vi "cumplimiento.vi"(8 "error in (no error)":errorcluster, 11 "Prueba08 in":refnum<class "Prueba32.lvclass">) -> (0 "error out":errorcluster, 1 "Evaluarcion Final":bool, 2 "cumpimiento":string, 3 "Prueba08 out":refnum<class "Prueba32.lvclass">)   [LabVIEW 2019, in "Prueba32.lvclass"]
uses:
  Prueba32.lvclass
  Prueba32.lvclass/Prueba32.ctl
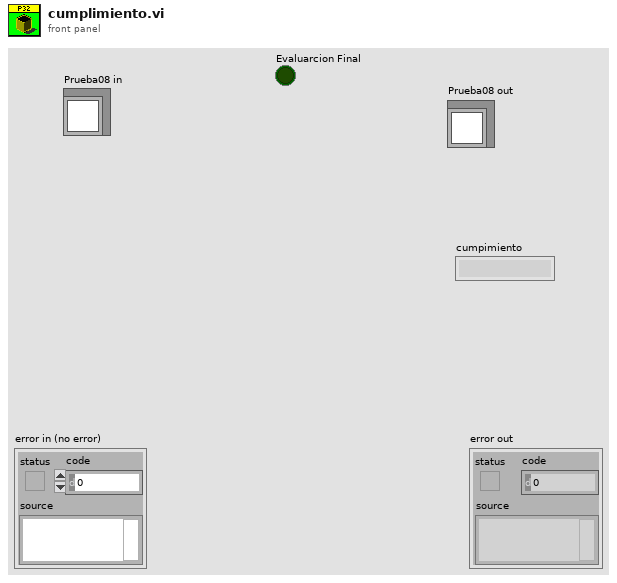
[diagram p1: front panel]
types:
  T1 = cluster{"Medido":dbl, "Error":dbl, "Ref":dbl, "Incert_exp":dbl, "Tol+":dbl, "Tol-":dbl, "fila":i32}
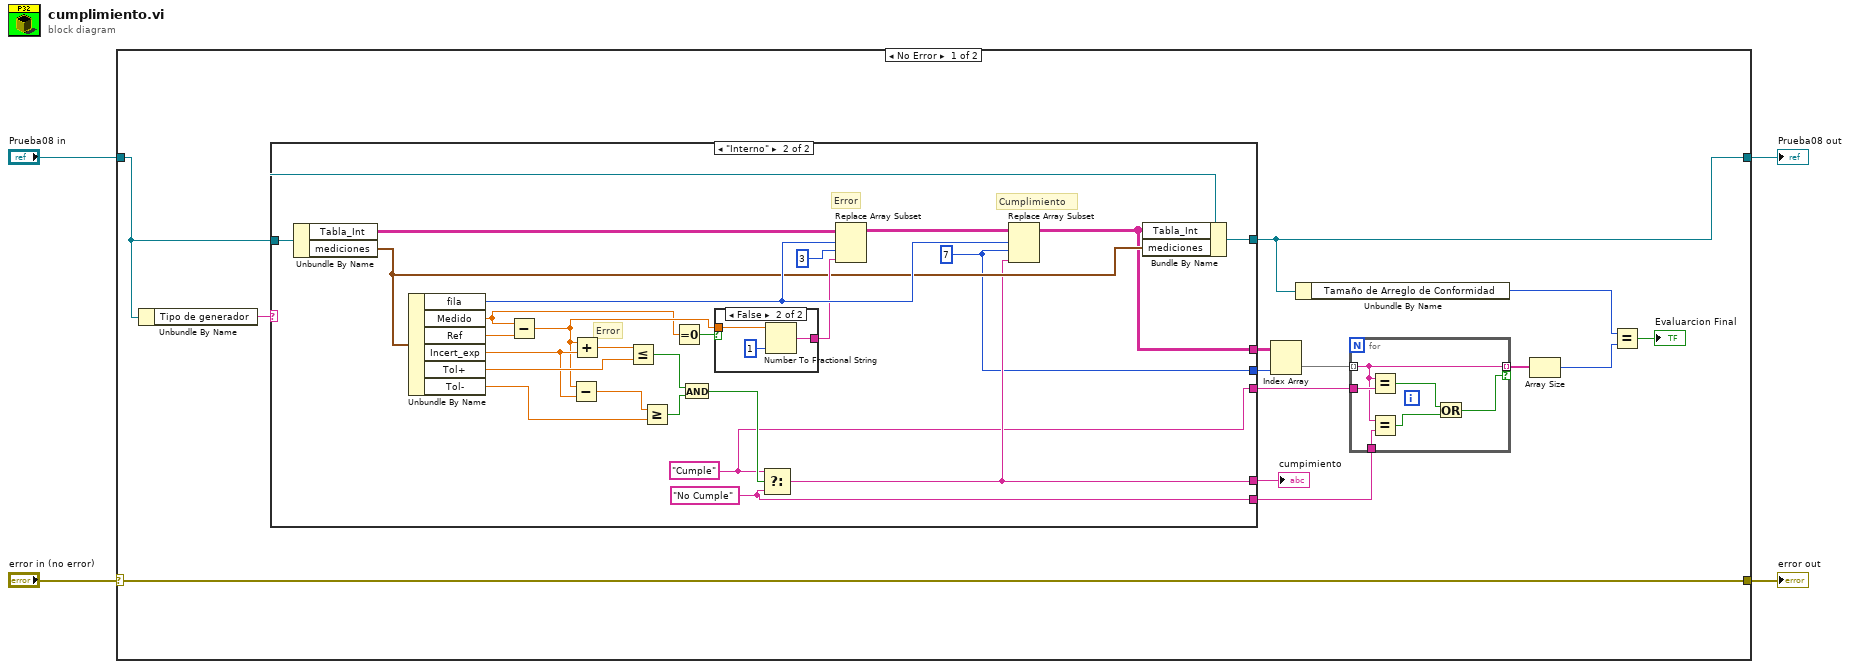
[diagram p0: block diagram]
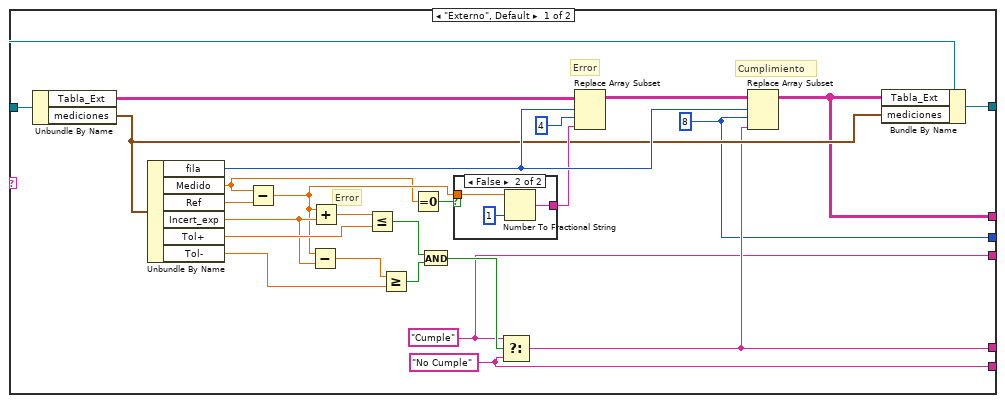
[diagram p2: hidden frame]
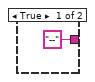
[diagram p3: hidden frame]
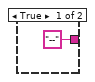
[diagram p4: hidden frame]
diagram:
  n1 = case shown="No Error" "error in (no error)" {
    selector: "error in (no error)" -> [w18 w84]
    tunnel: [w18 w84] -> w3
    tunnel: [w12 w83] -> w2
    tunnel: "Prueba08 in" -> [w17 w83]
    frame No Error {
      n2 = Unbundle By Name(w17) -> ("Tipo de generador"=w16:string)
      n3 = case shown="\"Interno\"" w16 {
        tunnel: [w34 w63] -> w12
        tunnel: w17 -> [w31 w60]
        tunnel: [w29 w58] -> w15
        tunnel: [w28 w57] -> w14
        tunnel: [w27 w56] -> w13
        tunnel: [w26 w55] -> w8
        tunnel: [w25 w54] -> w7
        frame "Externo", Default {
          w27 = 8 ("index (row)")
          w25 = "No Cumple"
          w26 = "Cumple"
          # "Cumplimiento"
          # "Error"
          # "Error"
          n4 = Unbundle By Name(w31) -> ("Tabla_Ext"=w33:string[][], "mediciones"=w32:T1)
          n5 = Unbundle By Name(w32) -> ("fila"=w40:i32, "Medido"=w35:dbl, "Ref"=w45:dbl, "Incert_exp"=w43:dbl, "Tol+"=w44:dbl, "Tol-"=w42:dbl)
          n6 = Subtract(x=w35, y=w45) -> (x-y=w36:dbl)
          n7 = Subtract(x=w36, y=w43) -> (x-y=w46:dbl)
          n8 = Add(x=w36, y=w43) -> (x+y=w49:dbl)
          n9 = Less Or Equal?(x=w49, y=w44) -> (x <= y?=w48:bool)
          n10 = Greater Or Equal?(x=w46, y=w42) -> (x >= y?=w47:bool)
          n11 = Equal To 0?(x=w35) -> (x = 0?=w37:bool)
          n12 = And(x=w48, y=w47) -> (x .and. y?=w30:bool)
          n13 = case shown="False" w37 {
            tunnel: w36 -> [_ w53]
            tunnel: ["--" w51] -> w38
            frame True {
            }
            frame False {
              n14 = Number To Fractional String(number=w53, precision (6)=i16 1) -> (F-format string=w51:string)  [unwired: 2 in]
            }
          }
          n15 = Select(t=w26, s=w30, f=w25) -> (s? t:f=w29:string)
          n16 = Replace Array Subset(array=w33, new element=w38, index (row)=w40, index (col)=4 ("disabled index (col)")) -> (w41:string[][])
          n17 = Replace Array Subset(array=w41, new element=w29, index (row)=w40, index (col)=w27) -> (w28:string[][])
          n18 = Bundle By Name(cluster=w31, "Tabla_Ext"=w28, "mediciones"=w32) -> (w34:refnum<class "Prueba32.lvclass">)
        }
        frame "Interno" {
          w56 = 7 ("index (row)")
          w54 = "No Cumple"
          w55 = "Cumple"
          # "Cumplimiento"
          # "Error"
          # "Error"
          n19 = Unbundle By Name(w60) -> ("Tabla_Int"=w62:string[][], "mediciones"=w61:T1)
          n20 = Unbundle By Name(w61) -> ("fila"=w69:i32, "Medido"=w64:dbl, "Ref"=w74:dbl, "Incert_exp"=w72:dbl, "Tol+"=w73:dbl, "Tol-"=w71:dbl)
          n21 = Subtract(x=w64, y=w74) -> (x-y=w65:dbl)
          n22 = Subtract(x=w65, y=w72) -> (x-y=w75:dbl)
          n23 = Add(x=w65, y=w72) -> (x+y=w78:dbl)
          n24 = Less Or Equal?(x=w78, y=w73) -> (x <= y?=w77:bool)
          n25 = Greater Or Equal?(x=w75, y=w71) -> (x >= y?=w76:bool)
          n26 = Equal To 0?(x=w64) -> (x = 0?=w66:bool)
          n27 = And(x=w77, y=w76) -> (x .and. y?=w59:bool)
          n28 = case shown="False" w66 {
            tunnel: w65 -> [_ w82]
            tunnel: ["--" w80] -> w67
            frame True {
            }
            frame False {
              n29 = Number To Fractional String(number=w82, precision (6)=i16 1) -> (F-format string=w80:string)  [unwired: 2 in]
            }
          }
          n30 = Select(t=w55, s=w59, f=w54) -> (s? t:f=w58:string)
          n31 = Replace Array Subset(array=w62, new element=w67, index (row)=w69, index (col)=3 ("disabled index (col)")) -> (w70:string[][])
          n32 = Replace Array Subset(array=w70, new element=w58, index (row)=w69, index (col)=w56) -> (w57:string[][])
          n33 = Bundle By Name(cluster=w60, "Tabla_Int"=w57, "mediciones"=w61) -> (w63:refnum<class "Prueba32.lvclass">)
        }
      }
      "cumpimiento" <- w15
      n34 = Index Array(array=w14, index (col)=w13) -> (element=w9:string[])  [unwired: 1 in]
      n35 = Unbundle By Name(w12) -> ("Tamaño de Arreglo de Conformidad"=w11:u16)
      n36 = for {
        tunnel: w9 -> [w20] mode=indexing
        tunnel: w8 -> [w24]
        tunnel: w7 -> [w22]
        tunnel: [w20] -> w6 mode=indexing if=w19
        n37 = Equal?(x=w20, y=w24) -> (x = y?=w23:bool)
        n38 = Equal?(x=w20, y=w22) -> (x = y?=w21:bool)
        n39 = Or(x=w23, y=w21) -> (x .or. y?=w19:bool)
      }
      n40 = Array Size(array=w6) -> (size(s)=w5:i32)
      n41 = Equal?(x=w11, y=w5) -> (x = y?=→"Evaluarcion Final":bool)
    }
    frame Error {
    }
  }
  "error out" <- w3
  "Prueba08 out" <- w2
